vi "Receive Messages.vi"(8 "error in":errorcluster, 10 "Sender":string, 11 "ICommunicate in":refnum<class "ICommunicate.lvclass">) -> (0 "error out":errorcluster, 2 "Messages":refnum<class "IMessage.lvclass">[](array[class]), 3 "ICommunicate out":refnum<class "ICommunicate.lvclass">)   [LabVIEW 2024, in "ICommunicate.lvclass"]
uses:
  ICommunicate.lvclass
  IMessage/IMessage.lvclass
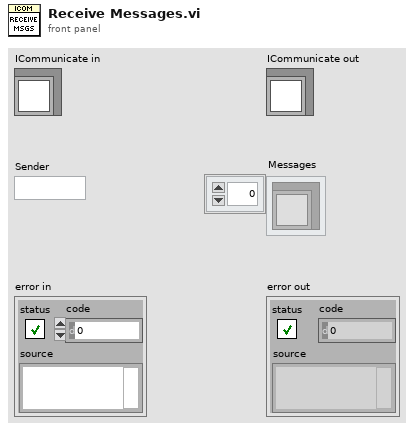
[diagram p1: front panel]
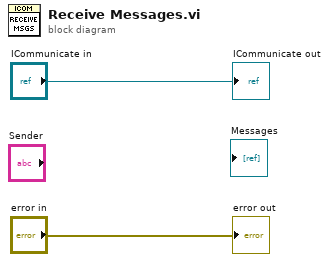
[diagram p0: block diagram]
diagram:
  "error out" <- "error in"
  "ICommunicate out" <- "ICommunicate in"
